vi "Sequencer Remote Control - Inbound&Outbound (Solution).vi"() -> ()   [LabVIEW 2019]
panel:
  out "Seq. Aborted?":bool
  out "Seq. Loaded?":bool
  out "Seq. Running?":bool
  out "AO Chart":cluster{"[0]":dbl, "[1]":dbl}(graph)
  in  "Run Sequence":bool
  in  "Load Sequence":bool
  in  "Sequence File Path":path
  in  "OK":bool
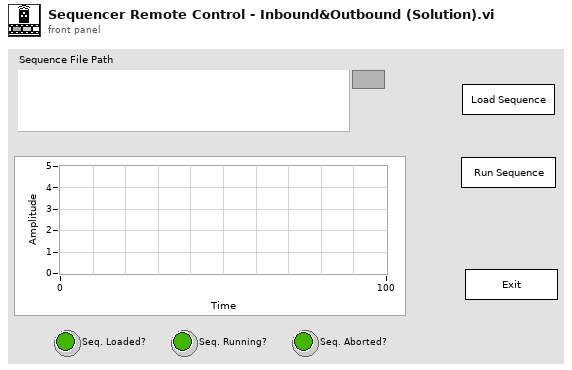
[diagram p1: front panel]
types:
  T1 = cluster{"Loaded":bool, "Running":bool, "Aborted":bool}
  T2 = cluster{"Sequencer Status":refnum<user-event>, "AO Data":refnum<user-event>}
  T3 = cluster{"Sequence File to Load":refnum<user-event>, "Run-Abort Sequence":refnum<user-event>, "Exit Sequencer":refnum<user-event>}
  T4 = enum32{"invalid app kind", "Development System", "Run Time System", "Student Edition", "Embedded LabVIEW", "Evaluation", "Custom"}
  T5 = enum32{"Invalid", "Standard", "Closed", "Hidden", "Minimized", "Maximized"}
  T6 = cluster{"Core":cluster{"Current VI Reference":refnum<vi>, "Close Panel on Exit?":bool}, "Inbound User Events":cluster{"Sequence File to Load":refnum<user-event>, "Run-Abort Sequence":refnum<user-event>, "Exit Sequencer":refnum<user-event>}, "Sequence File Path":path, "Outbound User Events":cluster{"Sequencer Status":refnum<user-event>, "AO Data":refnum<user-event>}, "Sequencer Status":cluster{"Loaded":bool, "Running":bool, "Aborted":bool}, "AO Data":cluster{"[0]":dbl, "[1]":dbl}}
  T7 = cluster{"Current VI Reference":refnum<vi>, "Close Panel on Exit?":bool}
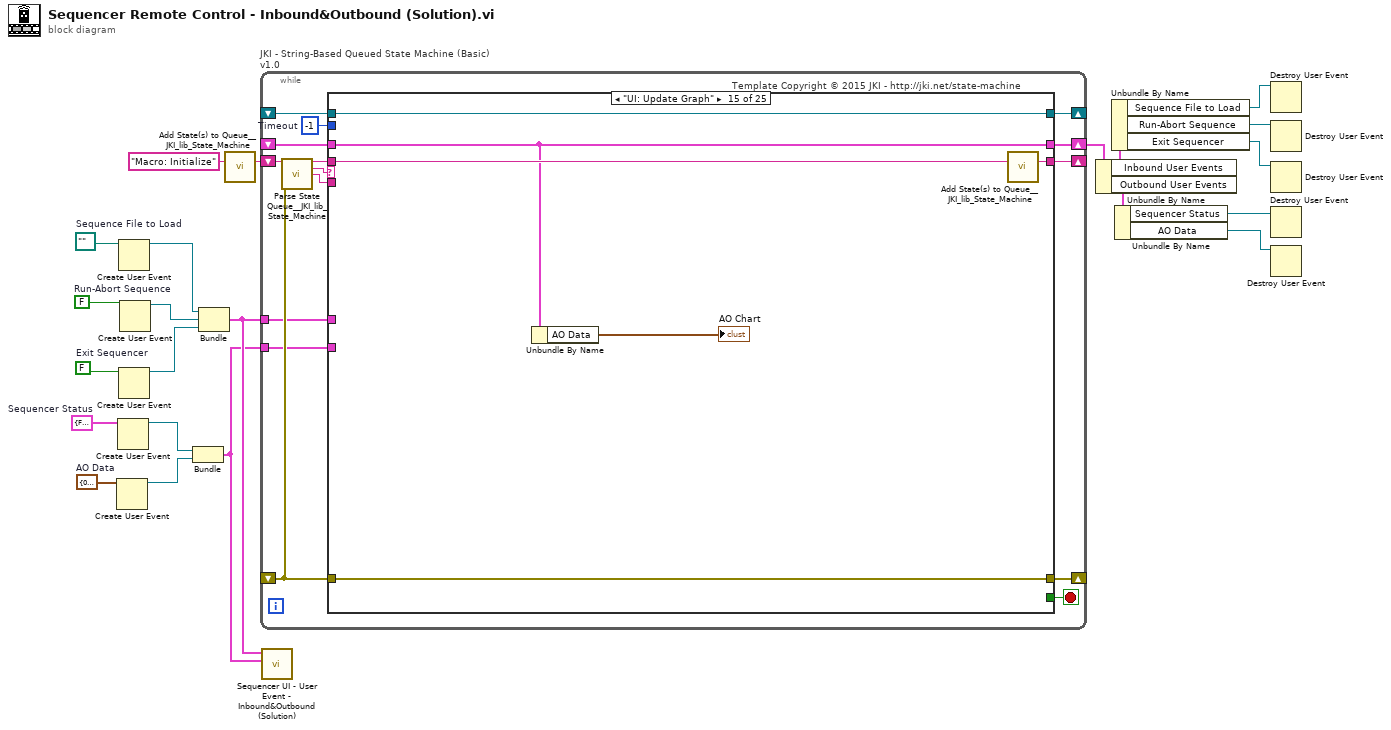
[diagram p0: block diagram]
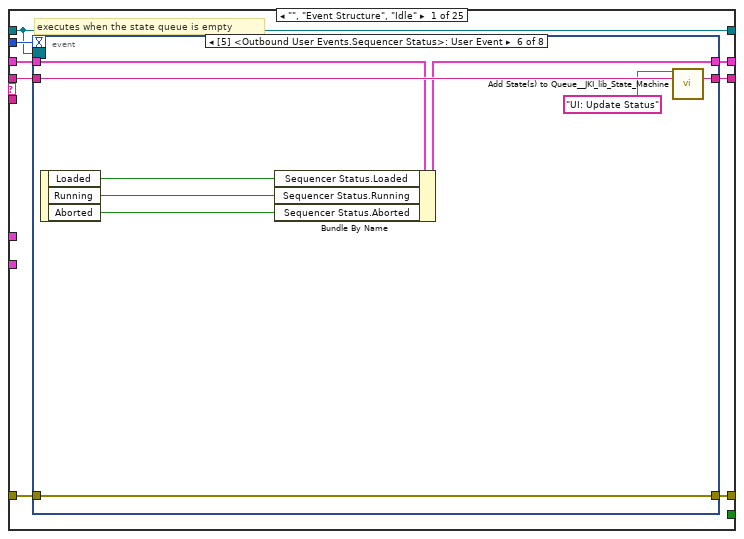
[diagram p2: hidden frame]
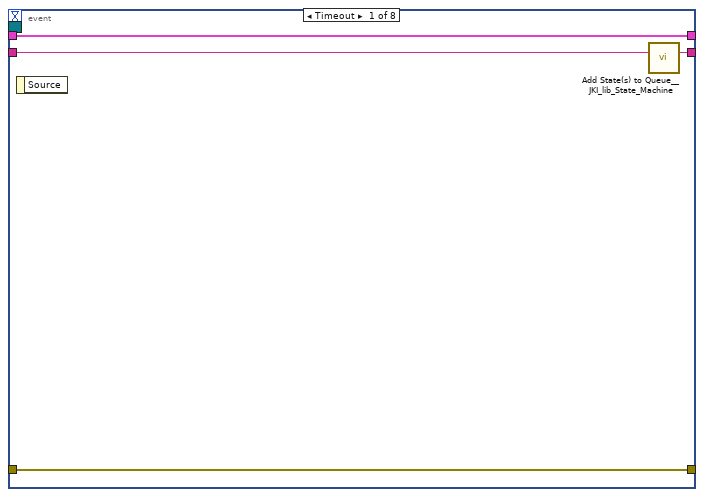
[diagram p3: hidden frame]
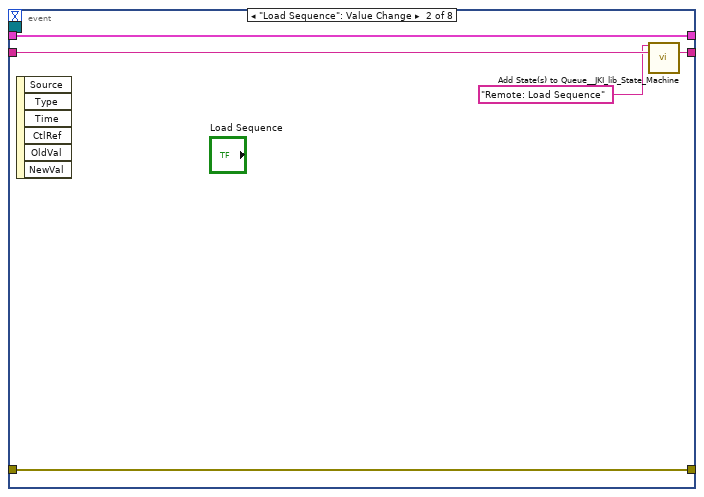
[diagram p4: hidden frame]
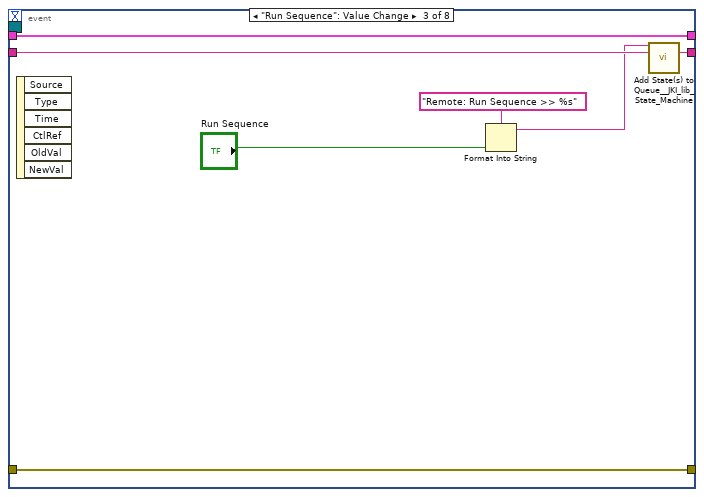
[diagram p5: hidden frame]
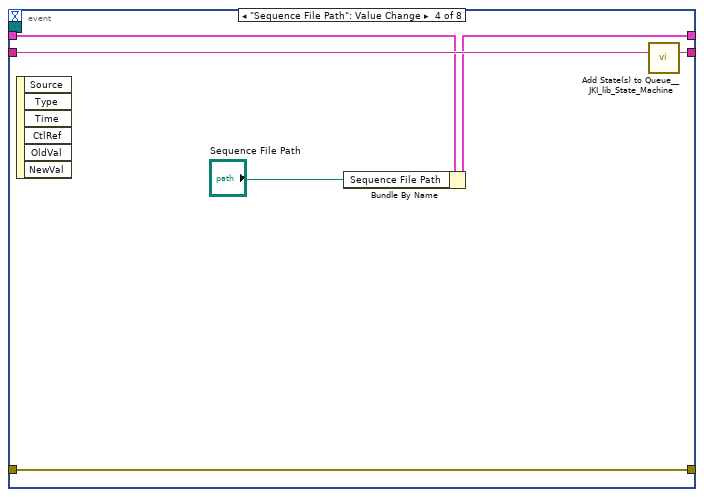
[diagram p6: hidden frame]
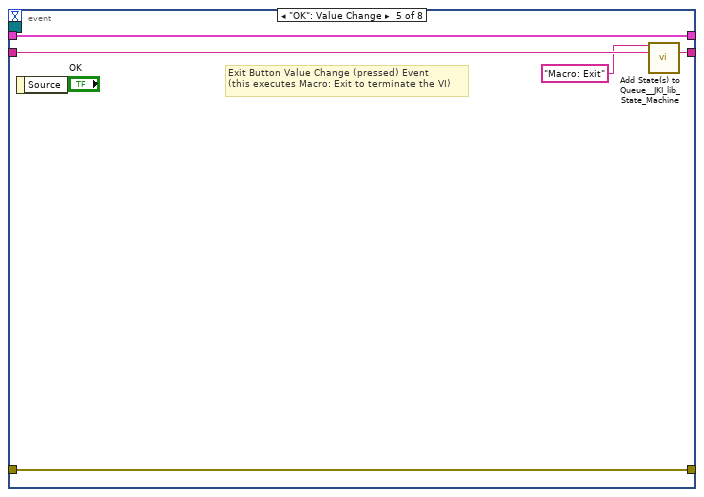
[diagram p7: hidden frame]
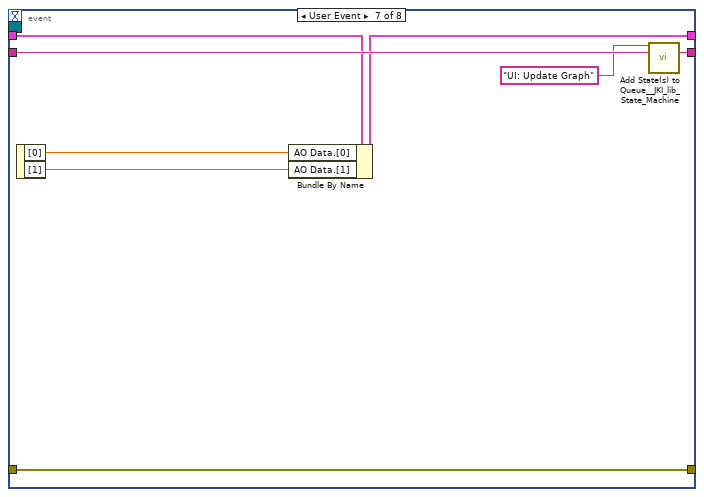
[diagram p8: hidden frame]
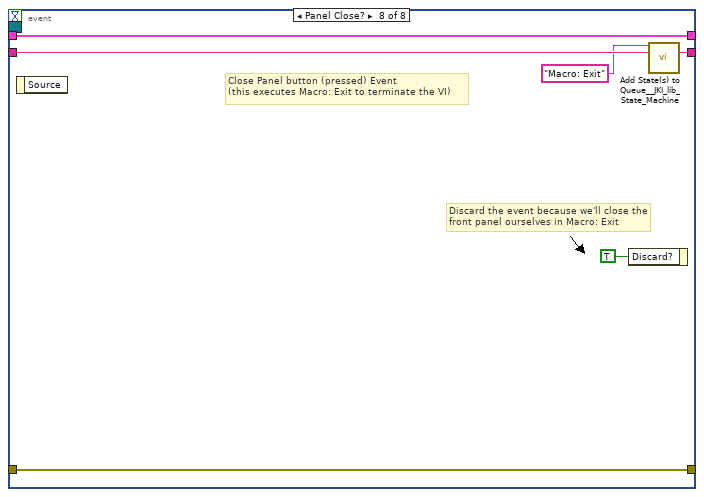
[diagram p9: hidden frame]
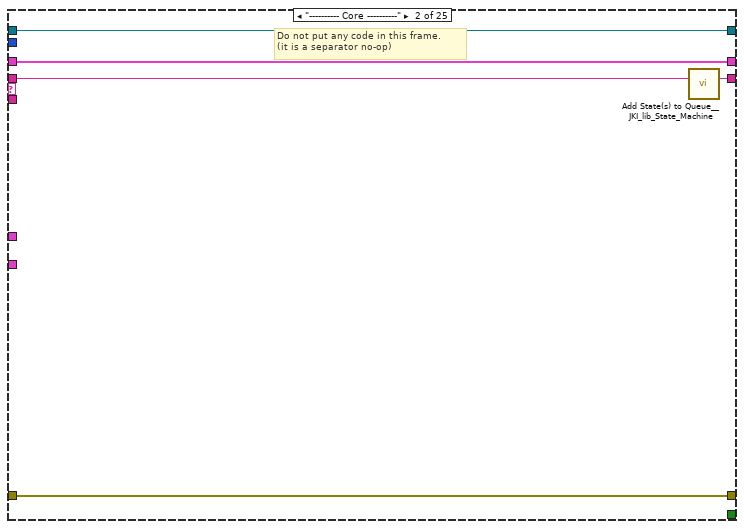
[diagram p10: hidden frame]
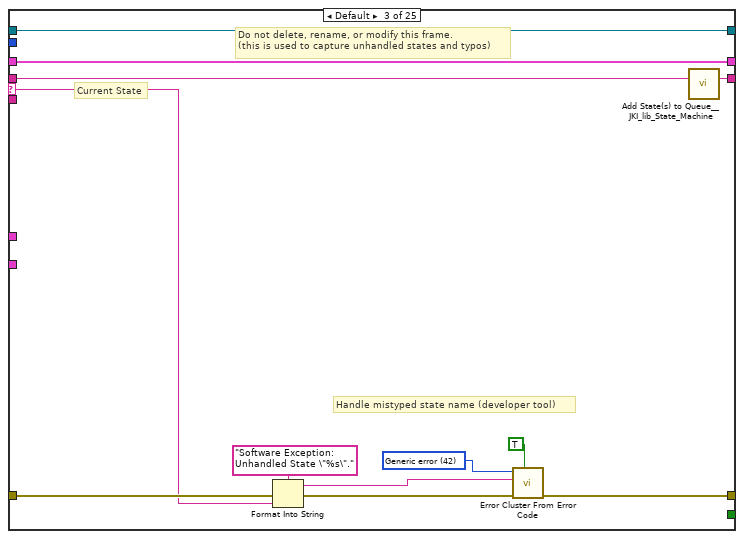
[diagram p11: hidden frame]
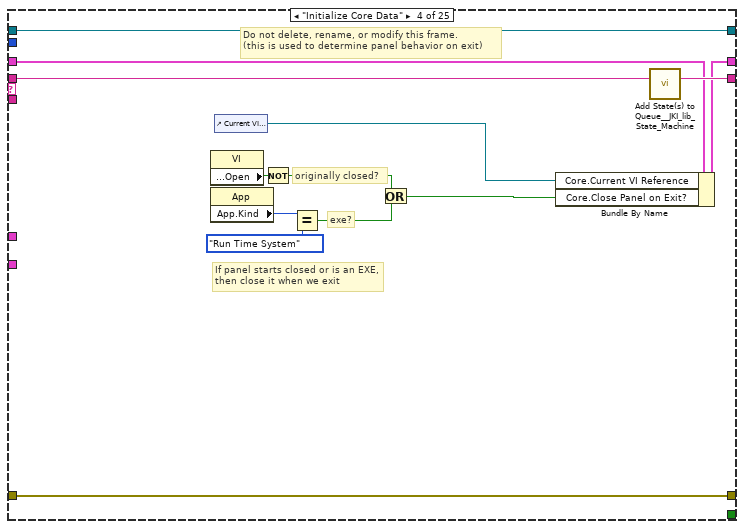
[diagram p12: hidden frame]
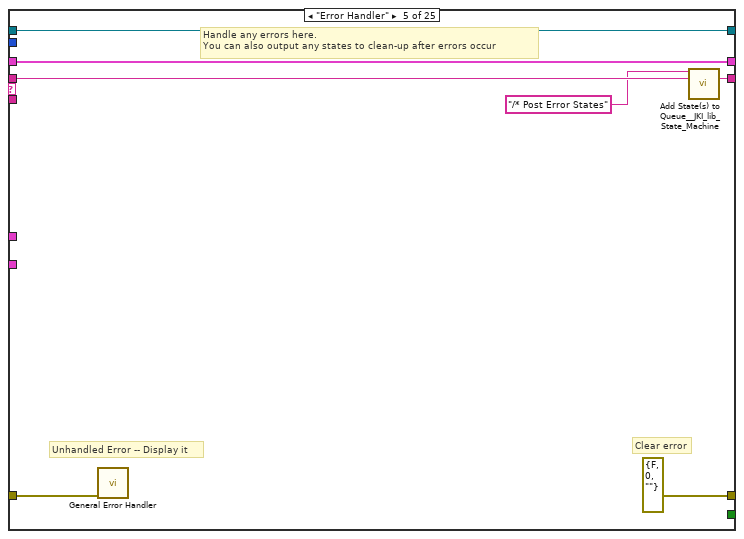
[diagram p13: hidden frame]
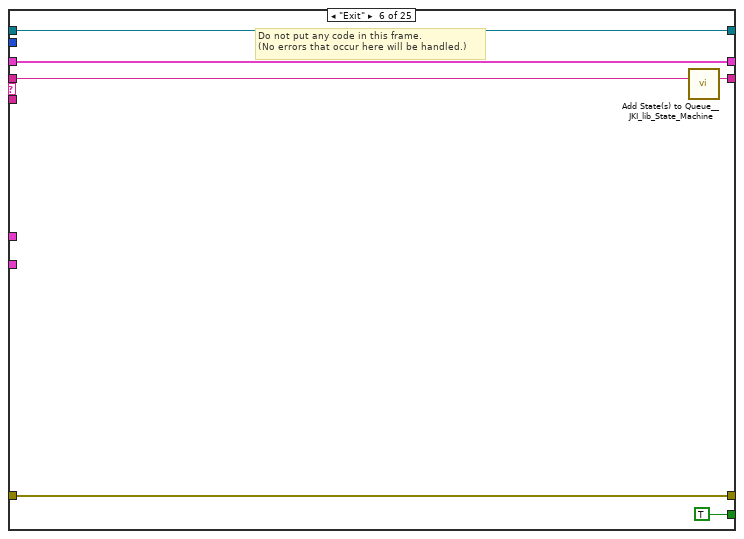
[diagram p14: hidden frame]
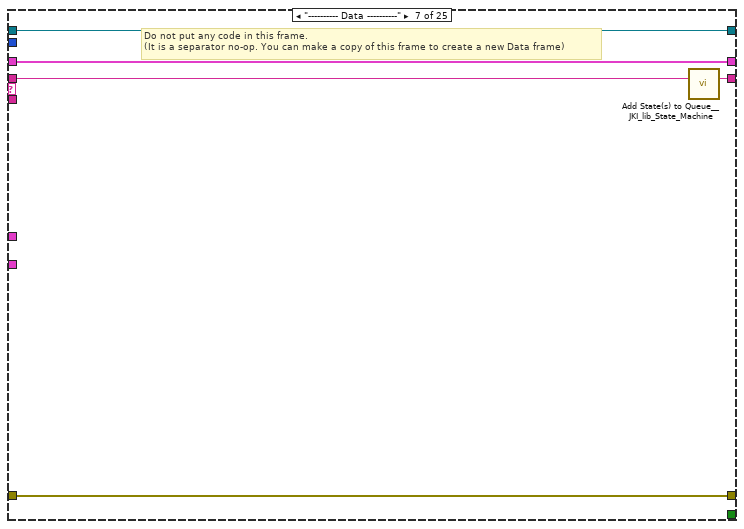
[diagram p15: hidden frame]
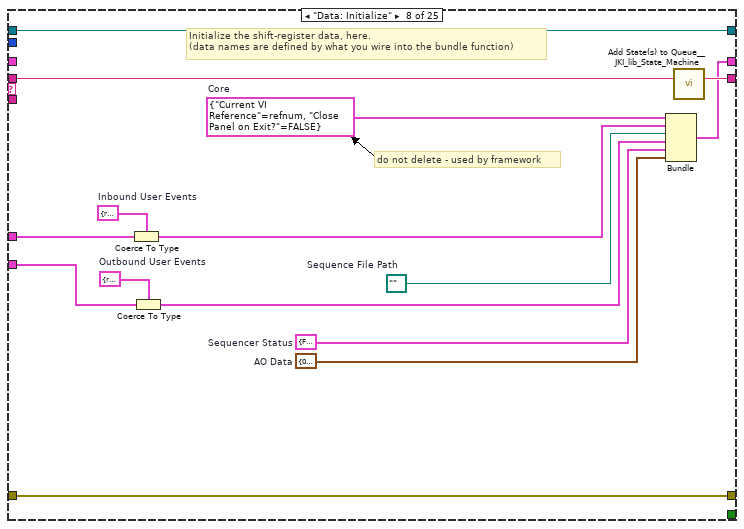
[diagram p16: hidden frame]
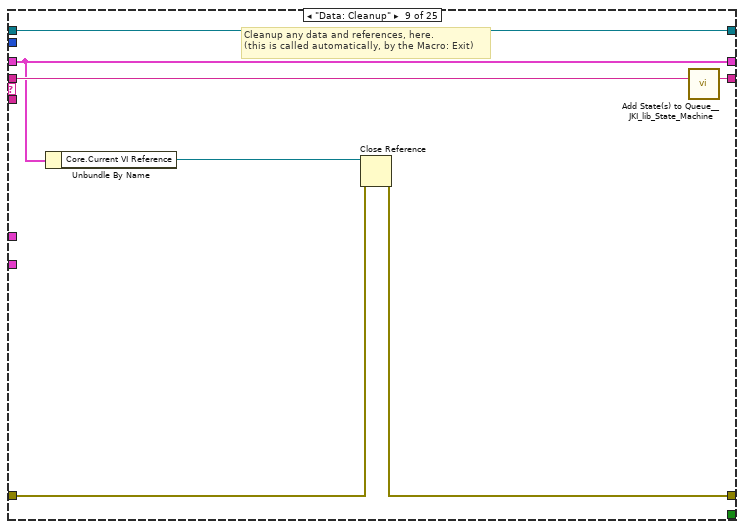
[diagram p17: hidden frame]
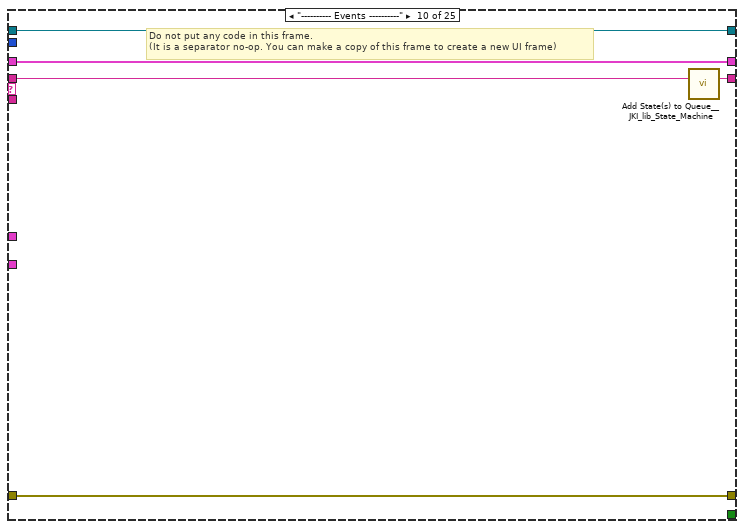
[diagram p18: hidden frame]
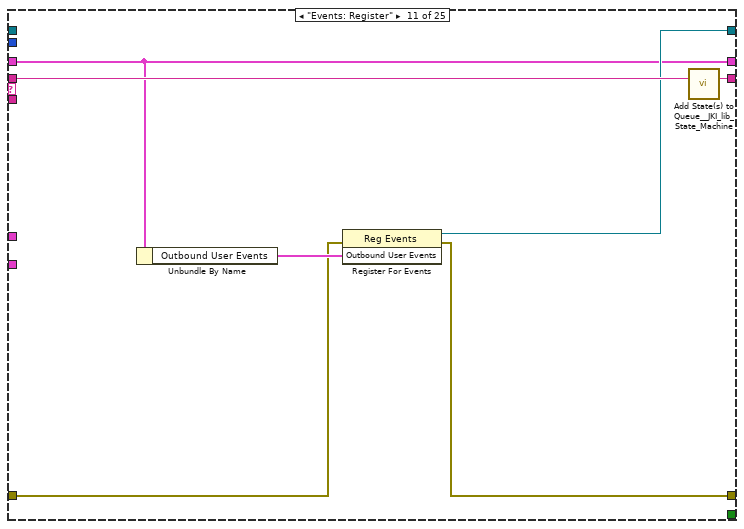
[diagram p19: hidden frame]
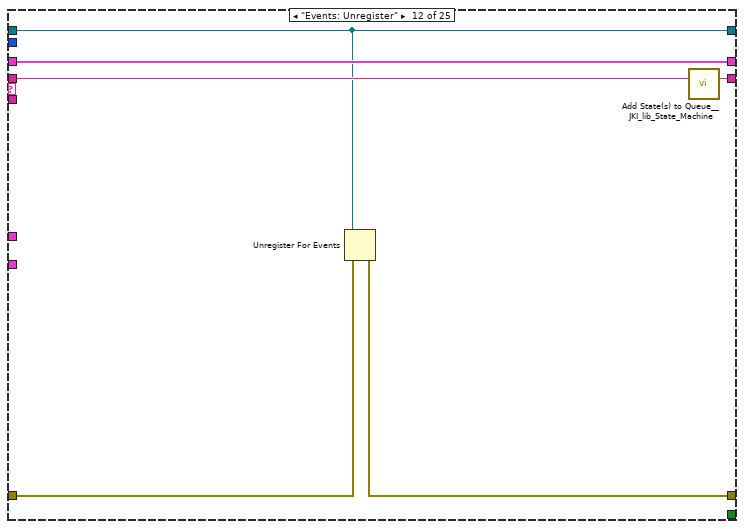
[diagram p20: hidden frame]
diagram:
  w7 = T1 {"Loaded"=FALSE, "Running"=FALSE, "Aborted"=FALSE}  # Sequencer Status
  w8 = cluster{"[0]":dbl, "[1]":dbl} {"[0]"=0.0, "[1]"=0.0}  # AO Data
  w18 = FALSE  # Exit Sequencer
  w19 = FALSE  # Run-Abort Sequence
  w20 = path ""  # Sequence File to Load
  n1 = Create User Event(user event datatype=w8) -> (user event=w5:refnum<user-event>)  [unwired: 1 in, 1 out]
  n2 = Create User Event(user event datatype=w7) -> (user event=w6:refnum<user-event>)  [unwired: 1 in, 1 out]
  n3 = Create User Event(user event datatype=w20) -> (user event=w17:refnum<user-event>)  [unwired: 1 in, 1 out]
  n4 = Create User Event(user event datatype=w18) -> (user event=w15:refnum<user-event>)  [unwired: 1 in, 1 out]
  n5 = Create User Event(user event datatype=w19) -> (user event=w16:refnum<user-event>)  [unwired: 1 in, 1 out]
  n6 = Bundle("Sequencer Status"=w6, "AO Data"=w5) -> (w4:T2)  [unwired: 1 in]
  n7 = Bundle("Sequence File to Load"=w17, "Run-Abort Sequence"=w16, "Exit Sequencer"=w15) -> (w9:T3)  [unwired: 1 in]
  n8 = call <vilib>:"Add State(s) to Queue__JKI_lib_State_Machine.vi"("State(s) in (\"\")"="Macro: Initialize") -> ("States Out"=w22:string)  [unwired: 14 in]
  n9 = while "JKI - String-Based Queued State Machine (Basic) v1.0" {
    shift-right: [w30] -> w14
    shift-left: _ -> [w29]
    shift-right: [w33] -> _
    shift-left: _ -> [w27]
    shift-right: [w32] -> _
    shift-left: w22 -> [w34]
    tunnel: w9 -> [w26]
    tunnel: w4 -> [w25]
    shift-right: [w24] -> _
    shift-left: _ -> [w23]
    stop <- w31 stop-if-true
    w28 = -1  # Timeout
    # "Template Copyright © 2015 JKI - http://jki.net/state-machine"
    n10 = call <vilib>:"Parse State Queue__JKI_lib_State_Machine.vi"("State Queue"=w34, "Error In (no error)"=w27) -> ("Remaining States"=w36:string, "Current State"=w37:string, "Arguments"=w35:string)  [unwired: 11 in]
    n11 = case shown="\"UI: Update Graph\"" w37 {
      selector: w37 -> [_ _ w102 _ _ _ _ _ _ _ _ _ _ _ _ _ _ _ _ _ _ _ _ _ _]
      tunnel: w36 -> [w45 w100 w106 w125 w132 w138 w143 w158 w165 w170 w177 w183 w188 w197 w204 w212 w219 w231 w258 w264 w276 w281 w289 w301 w309]
      tunnel: w35 -> [_ _ _ _ _ _ _ _ _ _ _ _ _ _ _ _ w214 w225 _ _ _ _ _ w297 _]
      tunnel: w29 -> [w43 w97 w104 w116 w129 w136 w140 _ w160 w167 w173 w181 w185 w193 w200 w207 w217 w227 w255 w261 w273 w278 w287 w298 w306]
      tunnel: [w42 w98 w108 w122 errorcluster {"status"=FALSE, "code"=0, "source"=""} ("error out") w135 w141 w155 w161 w168 w174 w178 w186 w195 w202 w210 w215 w228 w256 w262 w274 w279 w284 w292 w305] -> w33
      tunnel: w27 -> [w41 w98 w107 w122 w128 w135 w141 w155 w162 w168 w171 w179 w186 w195 w202 w210 w216 w229 w256 w262 w274 w279 w283 w291 w304]
      tunnel: [w44 w99 w105 w124 w131 w137 w142 w157 w164 w169 w176 w182 w187 w196 w203 w211 w218 w230 w257 w263 w275 w280 w288 w300 w308] -> w32
      tunnel: [_ _ _ _ _ TRUE _ _ _ _ _ _ _ _ _ _ _ _ _ _ _ _ _ _ _] -> w31
      tunnel: [w40 w97 w104 w123 w129 w136 w140 w156 w160 w167 w173 w181 w185 w193 w200 w207 w217 w227 w255 w261 w273 w278 w287 w298 w306] -> w30
      tunnel: w28 -> [w39 _ _ _ _ _ _ _ _ _ _ _ _ _ _ _ _ _ _ _ _ _ _ _ _]
      tunnel: w26 -> [_ _ _ _ _ _ _ w153 _ _ _ _ _ _ _ _ _ _ _ _ _ _ _ _ _]
      tunnel: w25 -> [_ _ _ _ _ _ _ w148 _ _ _ _ _ _ _ _ _ _ _ _ _ _ _ _ _]
      tunnel: [w38 w96 w101 w113 w126 w133 w139 w146 w159 w166 w175 w180 w184 w194 w201 w209 w213 w224 w254 w259 w265 w277 w282 w290 w302] -> w24
      tunnel: w23 -> [w38 w96 w101 w113 w126 w133 w139 w146 w159 w166 _ w180 w184 w194 w201 w209 w213 w224 w254 w259 w265 w277 w282 w290 w302]
      frame "", "Event Structure", "Idle" {
        # "executes when the state queue is empty"
        n12 = event shown="[5] <Outbound User Events.Sequencer Status>: User Event" {
          selector: w38 -> [_ _ _ _ _ _ _ _]
          dyn-events: _ -> [_ _ _ _ _ _ _ _]
          timeout: w39 -> [_ _ _ _ _ _ _ _]
          tunnel: w45 -> [w49 w54 w61 w67 w72 w81 w89 w95]
          tunnel: [w48 w53 w60 w66 w71 w80 w88 w94] -> w44
          tunnel: w43 -> [w46 w51 w58 w64 w69 w76 w84 w92]
          tunnel: [w47 w52 w59 w65 w70 w79 w87 w93] -> w42
          tunnel: w41 -> [w47 w52 w59 w65 w70 w79 w87 w93]
          tunnel: [w46 w51 w58 w63 w69 w77 w85 w92] -> w40
          event Timeout {
            n13 = event-data() -> ()  [unwired: 1 in, 1 out]
            n14 = call <vilib>:"Add State(s) to Queue__JKI_lib_State_Machine.vi"("State(s) in (\"\")"=w49) -> ("States Out"=w48:string)  [unwired: 14 in]
          }
          event "Load Sequence": Value Change {
            n15 = event-data() -> ()  [unwired: 1 in, 6 out]
            n16 = call <vilib>:"Add State(s) to Queue__JKI_lib_State_Machine.vi"("State(s) in Front (\"\")"="Remote: Load Sequence", "State(s) in (\"\")"=w54) -> ("States Out"=w53:string)  [unwired: 13 in]
          }
          event "Run Sequence": Value Change {
            n17 = event-data() -> ()  [unwired: 1 in, 6 out]
            n18 = Format Into String(format string="Remote: Run Sequence >> %s", "Run Sequence") -> (resulting string=w55:string)  [unwired: 2 in, 1 out]
            n19 = call <vilib>:"Add State(s) to Queue__JKI_lib_State_Machine.vi"("State(s) in Front (\"\")"=w55, "State(s) in (\"\")"=w61) -> ("States Out"=w60:string)  [unwired: 13 in]
          }
          event "Sequence File Path": Value Change {
            n20 = event-data() -> ()  [unwired: 1 in, 6 out]
            n21 = Bundle By Name(cluster=w64, "Sequence File Path"="Sequence File Path") -> (w63:T6)
            n22 = call <vilib>:"Add State(s) to Queue__JKI_lib_State_Machine.vi"("State(s) in (\"\")"=w67) -> ("States Out"=w66:string)  [unwired: 14 in]
          }
          event "OK": Value Change {
            # "Exit Button Value Change (pressed) Event\n(this executes Macro: Exit to terminate the VI)"
            n23 = event-data() -> ()  [unwired: 1 in, 1 out]
            n24 = call <vilib>:"Add State(s) to Queue__JKI_lib_State_Machine.vi"("State(s) in Front (\"\")"="Macro: Exit", "State(s) in (\"\")"=w72) -> ("States Out"=w71:string)  [unwired: 13 in]
          }
          event User Event {
            n25 = event-data() -> ("Loaded"=w75:bool, "Running"=w74:bool, "Aborted"=w73:bool)  [unwired: 1 in]
            n26 = Bundle By Name(cluster=w76, "Sequencer Status.Loaded"=w75, "Sequencer Status.Running"=w74, "Sequencer Status.Aborted"=w73) -> (w77:T6)
            n27 = call <vilib>:"Add State(s) to Queue__JKI_lib_State_Machine.vi"("State(s) in Front (\"\")"="UI: Update Status", "State(s) in (\"\")"=w81) -> ("States Out"=w80:string)  [unwired: 13 in]
          }
          event User Event {
            n28 = event-data() -> ("[0]"=w83:dbl, "[1]"=w82:dbl)  [unwired: 1 in]
            n29 = Bundle By Name(cluster=w84, "AO Data.[0]"=w83, "AO Data.[1]"=w82) -> (w85:T6)
            n30 = call <vilib>:"Add State(s) to Queue__JKI_lib_State_Machine.vi"("State(s) in Front (\"\")"="UI: Update Graph", "State(s) in (\"\")"=w89) -> ("States Out"=w88:string)  [unwired: 13 in]
          }
          event Panel Close? {
            # "Discard the event because we'll close the front panel ourselves in Macro: Exit"
            # "Close Panel button (pressed) Event\n(this executes Macro: Exit to terminate the VI)"
            n31 = event-data() -> ()  [unwired: 1 in, 1 out]
            n32 = event-data("Discard?"=TRUE) -> ()  [unwired: 1 in, 1 out]
            n33 = call <vilib>:"Add State(s) to Queue__JKI_lib_State_Machine.vi"("State(s) in Front (\"\")"="Macro: Exit", "State(s) in (\"\")"=w95) -> ("States Out"=w94:string)  [unwired: 13 in]
          }
        }
      }
      frame "---------- Core ----------" {
        # "Do not put any code in this frame.\n(it is a separator no-op)"
        n34 = call <vilib>:"Add State(s) to Queue__JKI_lib_State_Machine.vi"("State(s) in (\"\")"=w100) -> ("States Out"=w99:string)  [unwired: 14 in]
      }
      frame Default {
        w111 = 42 items=["No error", "Argument error", "Memory is full", "Out of zone", "End of file", "File already open", "Generic file I/O error", "File not found", "File permission error", "Disk is full", "Duplicate path", "Too many files open", "System feature not enabled", "Resource file not found", "Cannot add resource", "Resource not found", "Image not found", "Image memory error", "Pen does not exist", "Config type invalid", "Config token not found", "Config parse error", "Config memory error", "Bad external code format", "Bad external code offset", "External code not present", "Null window", "Destroy window error", "Null menu", "Print aborted", "Bad print record", "Print driver error", "Windows error during printing", "Memory error during printing", "Print dialog error", "Generic print error", "Invalid device refnum", "Device not found", "Device parameter error", "Device unit error", "Cannot open device", "Device call aborted", "Generic error", "Cancelled by user", "Object ID too low", "Object ID too high", "Object not in heap", "Unknown heap", "Unknown object (invalid DefProc)", "Unknown object (DefProc not in table)", "Message out of range", "Invalid (null) method", "Unknown message", "Manager call not supported", "Bad address", "Network operation in progress", "Network operation timed out", "Connection is busy", "Network attribute not supported", "Network error", "Address in use", "System out of memory", "Connection aborted", "Connection refused", "Not connected", "Already connected", "Connection closed", "Initialization error (interapplication manager)", "Bad occurrence", "Wait on unbound occurrence handler", "Occurrence queue overflow", "Datalog type conflict", "Unused", "Unrecognized type (interapplication manager)", "Memory corrupt", "Failed to make temporary DLL", "Old CIN version", "Drag socket not found", "Failed to load drop-object", "Failed to register OLE object", "Failed to release OLE object", "Format specifier type mismatch", "Unknown format specifier", "Too few format specifiers", "Too many format specifiers", "Scan failed", "Newer CIN version", "Error converting to variant", "Runtime menu error", "Password tampered", "Variant attribute not found", "Incompatible variant data type", "Event data is not available", "Event Store is not present", "Occurrence is not found", "Event Queue is not created", "Event info is not available", "Refnum passed is NULL", "Error retrieving Class GUID", "Error retrieving CoClass GUID", "Error retrieving TypeLib GUID.", "Bad built application magic bytes.", "Specific driver is different from the specific driver associated with the Logical Name.", "There is no session opened to the class driver.", "Max Error", "MAX - Error with config objects", "MAX - Error loading configuration", "MAX - Group not supported"]
        # "Current State"
        # "Do not delete, rename, or modify this frame.\n(this is used to capture unhandled states and typos)"
        # "Handle mistyped state name (developer tool)"
        n35 = Format Into String(format string="Software Exception: Unhandled State \"%s\"." ("message"), error in=w107, w102) -> (resulting string=w110:string, error out=w109:errorcluster)  [unwired: 1 in]
        n36 = call <vilib>:"Error Cluster From Error Code.vi"("show call chain? (False)"=TRUE, "error in (no error)"=w109, "error message (\"\")"=w110, "error code (0)"=w111) -> ("error out"=w108:errorcluster)  [unwired: 5 in]
        n37 = call <vilib>:"Add State(s) to Queue__JKI_lib_State_Machine.vi"("State(s) in (\"\")"=w106) -> ("States Out"=w105:string)  [unwired: 14 in]
      }
      frame "Initialize Core Data" {
        # "Do not delete, rename, or modify this frame.\n(this is used to determine panel behavior on exit)"
        # "originally closed?"
        # "exe?"
        # "If panel starts closed or is an EXE, then close it when we exit"
        n38 = property class="VI"() -> ("Front Panel.Open"=w121:bool)  [unwired: 2 in, 2 out]
        n39 = property class="App"() -> ("App.Kind"=w120:T4)  [unwired: 2 in, 2 out]
        n40 = control-ref of="Current VI Reference"() -> (w114:refnum<vi>)
        n41 = Not(x=w121) -> (.not. x?=w118:bool)
        n42 = Equal?(x=w120, y=T4."Run Time System" ("Application:Kind")) -> (x = y?=w117:bool)
        n43 = Or(x=w118, y=w117) -> (x .or. y?=w115:bool)
        n44 = Bundle By Name(cluster=w116, "Core.Current VI Reference"=w114, "Core.Close Panel on Exit?"=w115) -> (w123:T6)
        n45 = call <vilib>:"Add State(s) to Queue__JKI_lib_State_Machine.vi"("State(s) in (\"\")"=w125) -> ("States Out"=w124:string)  [unwired: 14 in]
      }
      frame "Error Handler" {
        # "Unhandled Error -- Display it"
        # "Handle any errors here.\nYou can also output any states to clean-up after errors occur"
        # "Clear error"
        n46 = call <vilib>:"General Error Handler.vi"("error in (no error)"=w128) -> ()  [unwired: 10 in, 5 out]
        n47 = call <vilib>:"Add State(s) to Queue__JKI_lib_State_Machine.vi"("State(s) in Front (\"\")"="/* Post Error States", "State(s) in (\"\")"=w132) -> ("States Out"=w131:string)  [unwired: 13 in]
      }
      frame "Exit" {
        # "Do not put any code in this frame.\n(No errors that occur here will be handled.)"
        n48 = call <vilib>:"Add State(s) to Queue__JKI_lib_State_Machine.vi"("State(s) in (\"\")"=w138) -> ("States Out"=w137:string)  [unwired: 14 in]
      }
      frame "---------- Data ----------" {
        # "Do not put any code in this frame.\n(It is a separator no-op. You can make a copy of this frame to create a new Data frame)"
        n49 = call <vilib>:"Add State(s) to Queue__JKI_lib_State_Machine.vi"("State(s) in (\"\")"=w143) -> ("States Out"=w142:string)  [unwired: 14 in]
      }
      frame "Data: Initialize" {
        w145 = T1 {"Loaded"=FALSE, "Running"=FALSE, "Aborted"=FALSE}  # Sequencer Status
        w144 = cluster{"[0]":dbl, "[1]":dbl} {"[0]"=0.0, "[1]"=0.0}  # AO Data
        w147 = T2 {"Sequencer Status"=refnum, "AO Data"=refnum}  # Outbound User Events
        w150 = T3 {"Sequence File to Load"=refnum, "Run-Abort Sequence"=refnum, "Exit Sequencer"=refnum}  # Inbound User Events
        w152 = path ""  # Sequence File Path
        w154 = T7 {"Current VI Reference"=refnum, "Close Panel on Exit?"=FALSE}  # Core
        # "do not delete - used by framework"
        # "Initialize the shift-register data, here.\n(data names are defined by what you wire into the bundle function)"
        n50 = Coerce To Type(0:w153, 1:w150) -> (2:w151:T3)
        n51 = Coerce To Type(0:w148, 1:w147) -> (2:w149:T2)
        n52 = Bundle("Core"=w154, "Inbound User Events"=w151, "Sequence File Path"=w152, "Outbound User Events"=w149, "Sequencer Status"=w145, "AO Data"=w144) -> (w156:T6)  [unwired: 1 in]
        n53 = call <vilib>:"Add State(s) to Queue__JKI_lib_State_Machine.vi"("State(s) in (\"\")"=w158) -> ("States Out"=w157:string)  [unwired: 14 in]
      }
      frame "Data: Cleanup" {
        # "Cleanup any data and references, here.\n(this is called automatically, by the Macro: Exit)"
        n54 = Unbundle By Name(w160) -> ("Core.Current VI Reference"=w163:refnum<vi>)
        n55 = Close Reference(reference=w163, error in (no error)=w162) -> (error out=w161:errorcluster)
        n56 = call <vilib>:"Add State(s) to Queue__JKI_lib_State_Machine.vi"("State(s) in (\"\")"=w165) -> ("States Out"=w164:string)  [unwired: 14 in]
      }
      frame "---------- Events ----------" {
        # "Do not put any code in this frame.\n(It is a separator no-op. You can make a copy of this frame to create a new UI frame)"
        n57 = call <vilib>:"Add State(s) to Queue__JKI_lib_State_Machine.vi"("State(s) in (\"\")"=w170) -> ("States Out"=w169:string)  [unwired: 14 in]
      }
      frame "Events: Register" {
        n58 = Unbundle By Name(w173) -> ("Outbound User Events"=w172:T2)
        n59 = register-events(error in=w171, w172) -> (reference out=w175:refnum<event-registration>, error out=w174:errorcluster)  [unwired: 1 in]
        n60 = call <vilib>:"Add State(s) to Queue__JKI_lib_State_Machine.vi"("State(s) in (\"\")"=w177) -> ("States Out"=w176:string)  [unwired: 14 in]
      }
      frame "Events: Unregister" {
        n61 = Unregister For Events(event registration refnum=w180, error in=w179) -> (error out=w178:errorcluster)
        n62 = call <vilib>:"Add State(s) to Queue__JKI_lib_State_Machine.vi"("State(s) in (\"\")"=w183) -> ("States Out"=w182:string)  [unwired: 14 in]
      }
      frame "---------- UI ----------" {
        # "Do not put any code in this frame.\n(It is a separator no-op. You can make a copy of this frame to create a new UI frame)"
        n63 = call <vilib>:"Add State(s) to Queue__JKI_lib_State_Machine.vi"("State(s) in (\"\")"=w188) -> ("States Out"=w187:string)  [unwired: 14 in]
      }
      frame "UI: Update Status" {
        n64 = Unbundle By Name(w193) -> ("Sequencer Status.Loaded"=→"Seq. Loaded?":bool, "Sequencer Status.Running"=w190:bool, "Sequencer Status.Aborted"=→"Seq. Aborted?":bool)
        "Seq. Running?" <- w190
        n65 = call <userlib>:"Boolean Trigger__ogtk.vi"("Boolean Input"=w190) -> ("Falling Edge"=w189:bool)  [unwired: 1 in, 1 out]
        n66 = case shown="True" w189 {
          frame False {
          }
          frame True {
            n67 = local write "Run Sequence"(FALSE ("Run Sequence")) -> ()
          }
        }
        n68 = call <vilib>:"Add State(s) to Queue__JKI_lib_State_Machine.vi"("State(s) in (\"\")"=w197) -> ("States Out"=w196:string)  [unwired: 14 in]
      }
      frame "UI: Update Graph" {
        n69 = Unbundle By Name(w200) -> ("AO Data"=→"AO Chart":cluster{"[0]":dbl, "[1]":dbl})
        n70 = call <vilib>:"Add State(s) to Queue__JKI_lib_State_Machine.vi"("State(s) in (\"\")"=w204) -> ("States Out"=w203:string)  [unwired: 14 in]
      }
      frame "UI: Initialize" {
        # "Initialize the User Interface, here.\n(this is called automatically, by the Macro: Init)"
        n71 = Unbundle By Name(w207) -> ("Sequence File Path"=w206:path)
        n72 = local write "Sequence File Path"(w206) -> ()
        n73 = local write "Run Sequence"(FALSE ("Run Sequence")) -> ()
        n74 = property on="AO Chart" class="WFChart (strict)"("History Data"=cluster{"[0]":dbl, "[1]":dbl}[] []) -> ()  [unwired: 2 in, 2 out]
        n75 = call <vilib>:"Add State(s) to Queue__JKI_lib_State_Machine.vi"("State(s) in (\"\")"=w212) -> ("States Out"=w211:string)  [unwired: 14 in]
      }
      frame "UI: Cursor Set" {
        # "Argument"
        # "Set and Unset Cursor Busy.\n(Usage: \"UI: Cursor Set >> Busy|Idle\")"
        n76 = case shown="\"Idle\", Default" w214 {
          tunnel: w216 -> [w221 w223]
          tunnel: [w220 w222] -> w215
          frame "Idle", Default {
            n77 = call <vilib>:"Unset Busy.vi"("error in (no error)"=w221) -> ("error out"=w220:errorcluster)  [unwired: 10 in]
          }
          frame "Busy" {
            n78 = call <vilib>:"Set Busy.vi"("error in (no error)"=w223) -> ("error out"=w222:errorcluster)  [unwired: 9 in, 1 out]
          }
        }
        n79 = call <vilib>:"Add State(s) to Queue__JKI_lib_State_Machine.vi"("State(s) in (\"\")"=w219) -> ("States Out"=w218:string)  [unwired: 14 in]
      }
      frame "UI: Front Panel State" {
        # "Argument"
        # "Set Front Panel Open or Closed\n(Usage: \"UI: Front Panel State >> Open|Close\")"
        n80 = Unbundle By Name(w227) -> ("Core.Current VI Reference"=w226:refnum<vi>)
        n81 = case shown="\"Open\", Default" w225 {
          tunnel: w229 -> [w235 w248]
          tunnel: [w237 w249] -> w228
          tunnel: w226 -> [w236 w246]
          frame "Open", Default {
            n82 = property class="VI"(reference=w236, error in=w235) -> (reference out=w233:refnum<vi>, error out=w234:errorcluster, "Front Panel.Open"=w232:bool)
            n83 = case shown="False" w232 {
              tunnel: [w240 w243] -> w237
              tunnel: w234 -> [w239 w243]
              tunnel: w233 -> [w238 _]
              frame False {
                n84 = invoke class="VI" method="FP.Open"(reference=w238, error in=w239, "Activate"=TRUE, "State"=T5."Standard") -> (error out=w240:errorcluster)  [unwired: 1 in, 4 out]
              }
              frame True {
              }
            }
          }
          frame "Close" {
            n85 = property class="VI"(reference=w246, error in=w248) -> (reference out=w245:refnum<vi>, error out=w247:errorcluster, "Front Panel.Open"=w244:bool)
            n86 = case shown="True" w244 {
              tunnel: [w250 w253] -> w249
              tunnel: w247 -> [w250 w252]
              tunnel: w245 -> [_ w251]
              frame False {
              }
              frame True {
                n87 = invoke class="VI" method="FP.Close"(reference=w251, error in=w252) -> (error out=w253:errorcluster)  [unwired: 1 in, 2 out]
              }
            }
          }
        }
        n88 = call <vilib>:"Add State(s) to Queue__JKI_lib_State_Machine.vi"("State(s) in (\"\")"=w231) -> ("States Out"=w230:string)  [unwired: 14 in]
      }
      frame "---------- Macro ----------" {
        # "Do not put any code in this frame.\n(It is a separator no-op. You can make a copy of this frame to create a new Macro frame)"
        n89 = call <vilib>:"Add State(s) to Queue__JKI_lib_State_Machine.vi"("State(s) in (\"\")"=w258) -> ("States Out"=w257:string)  [unwired: 14 in]
      }
      frame "Macro: Initialize" {
        # "Initialization Macro\n(This is called once, when the VI starts)"
        n90 = call <vilib>:"Add State(s) to Queue__JKI_lib_State_Machine.vi"("State(s) in Front (\"\")"="Data: Initialize\nInitialize Core Data\nEvents: Register\nUI: Initialize\nUI: Update Status\nUI: Front Panel State >> Open", "State(s) in (\"\")"=w264) -> ("States Out"=w263:string)  [unwired: 13 in]
      }
      frame "Macro: Exit" {
        # "Exit Macro\n(This is called once, when the VI exits)"
        n91 = Unbundle By Name(w273) -> ("Core.Close Panel on Exit?"=w272:bool)
        n92 = Select(t="UI: Front Panel State >> Close", s=w272, f="") -> (s? t:f=w269:string)
        n93 = call <vilib>:"Add State(s) to Queue__JKI_lib_State_Machine.vi"("State(s) in Front (\"\")"="Remote: Exit Sequencer", "State(s) in (\"\")"=w269, "State(s) at Back (\"\")"="Data: Cleanup\nEvents: Unregister\nExit") -> ("States Out"=w267:string)  [unwired: 12 in]
        n94 = call <vilib>:"Add State(s) to Queue__JKI_lib_State_Machine.vi"("State(s) in Front (\"\")"=w267, "State(s) in (\"\")"=w276) -> ("States Out"=w275:string)  [unwired: 13 in]
      }
      frame "---------- Remote ----------" {
        # "Template Separator\n(You can make a copy of, or modify, this frame)"
        n95 = call <vilib>:"Add State(s) to Queue__JKI_lib_State_Machine.vi"("State(s) in (\"\")"=w281) -> ("States Out"=w280:string)  [unwired: 14 in]
      }
      frame "Remote: Load Sequence" {
        n96 = Unbundle By Name(w287) -> ("Inbound User Events.Sequence File to Load"=w286:refnum<user-event>, "Sequence File Path"=w285:path)
        n97 = Generate User Event(user event=w286, event data cluster=w285, error in=w283) -> (error out=w284:errorcluster)  [unwired: 1 in, 1 out]
        n98 = call <vilib>:"Add State(s) to Queue__JKI_lib_State_Machine.vi"("State(s) in (\"\")"=w289) -> ("States Out"=w288:string)  [unwired: 14 in]
      }
      frame "Remote: Run Sequence" {
        # "Remote: Run Sequence >> TRUE  //RUN\nRemote: Run Sequence >> FALSE //ABORT"
        n99 = Unbundle By Name(w298) -> ("Inbound User Events.Run-Abort Sequence"=w299:refnum<user-event>)
        n100 = To Upper Case(1:"TRUE" ("y")) -> (0:w293:string)
        n101 = To Upper Case(1:w297) -> (0:w294:string)
        n102 = Equal?(x=w294, y=w293) -> (x = y?=w295:bool)
        n103 = Generate User Event(user event=w299, event data cluster=w295, error in=w291) -> (error out=w292:errorcluster)  [unwired: 1 in, 1 out]
        n104 = call <vilib>:"Add State(s) to Queue__JKI_lib_State_Machine.vi"("State(s) in (\"\")"=w301) -> ("States Out"=w300:string)  [unwired: 14 in]
      }
      frame "Remote: Exit Sequencer" {
        n105 = Unbundle By Name(w306) -> ("Inbound User Events.Exit Sequencer"=w307:refnum<user-event>)
        n106 = Generate User Event(user event=w307, event data cluster=TRUE ("event data"), error in=w304) -> (error out=w305:errorcluster)  [unwired: 1 in, 1 out]
        n107 = call <vilib>:"Add State(s) to Queue__JKI_lib_State_Machine.vi"("State(s) in (\"\")"=w309) -> ("States Out"=w308:string)  [unwired: 14 in]
      }
    }
  }
  n108 = call "Sequencer UI - User Event - Inbound&Outbound (Solution).vi"("Outbound User Events"=w4, "Inbound User Events"=w9) -> ()  [unwired: 10 in]
  n109 = Unbundle By Name(w14) -> ("Inbound User Events"=w13:T3, "Outbound User Events"=w1:T2)
  n110 = Unbundle By Name(w13) -> ("Sequence File to Load"=w12:refnum<user-event>, "Run-Abort Sequence"=w11:refnum<user-event>, "Exit Sequencer"=w10:refnum<user-event>)
  n111 = Unbundle By Name(w1) -> ("Sequencer Status"=w2:refnum<user-event>, "AO Data"=w3:refnum<user-event>)
  n112 = Destroy User Event(user event=w12) -> ()  [unwired: 1 in, 1 out]
  n113 = Destroy User Event(user event=w11) -> ()  [unwired: 1 in, 1 out]
  n114 = Destroy User Event(user event=w10) -> ()  [unwired: 1 in, 1 out]
  n115 = Destroy User Event(user event=w2) -> ()  [unwired: 1 in, 1 out]
  n116 = Destroy User Event(user event=w3) -> ()  [unwired: 1 in, 1 out]
